vi "Test PWM host.vi"() -> ()   [LabVIEW 2013]
uses:
  <vilib>/userdefined/High Color/nirio_resource_hc.ctl
  <vilib>/rvi/interface/common/niFpgaWaitOnOcc.vi
  <vilib>/FPGAPlugInAG/PCIe-1473R/niLvFpga_Open_PCIe-1473R.vi
  <vilib>/rvi/interface/common/dynamic/niFpgaDynamicAddResources.vi
  <vilib>/Utility/error.llb/Error Cluster From Error Code.vi
  <vilib>/rvi/errors/niLvFpgaAdjustHostInterfaceError.vi
  <vilib>/FPGAPlugInAG/Dynamic/niLvFpga_Close_Dynamic.vi
  <vilib>/rvi/interface/nirviOpenFPGA/nirviOpenFPGA.xnode
  FPGA Bitfiles/PWMTest.lvbitx
  FPGA VIs/PWM FPGA test.vi
  <vilib>/rvi/interface/nirviReadWriteControl/nirviReadWriteControl.xnode
  <vilib>/rvi/interface/nirviCloseFPGA/nirviCloseFPGA.xnode
  NiFpgaLv.dll
  <vilib>/rvi/interface/Simulation/niFpgaSimulationCallBeginRW.vi
panel:
  in  "TTL 1":bool=TRUE
  in  "TTL 2":bool=TRUE
  in  "ISO Out 2":bool
  in  "ISO Out 1":bool
  in  "ISO Out 0":bool
  in  "resource name":T1="rio0" caption="RIO Device"
  out "error out":errorcluster
  out "Running?":bool
  in  "Stop":bool
  in  "Carrier Frequency (Hz)":dbl(slide)=1000.0 scale=0.0..10000000.0 scale format="%#_6p"
  in  "Duty cycle":dbl(slide)=0.5 scale=0.0..1.0
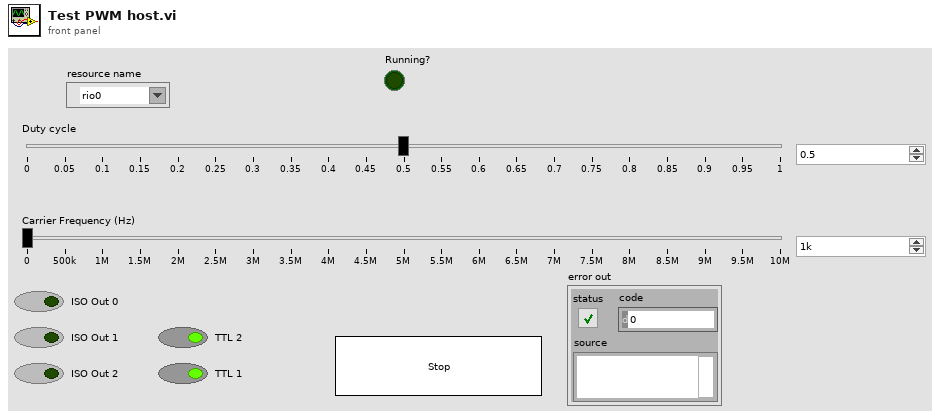
[diagram p1: front panel]
types:
  T1 = typedef "nirio_resource_hc.ctl" = tag
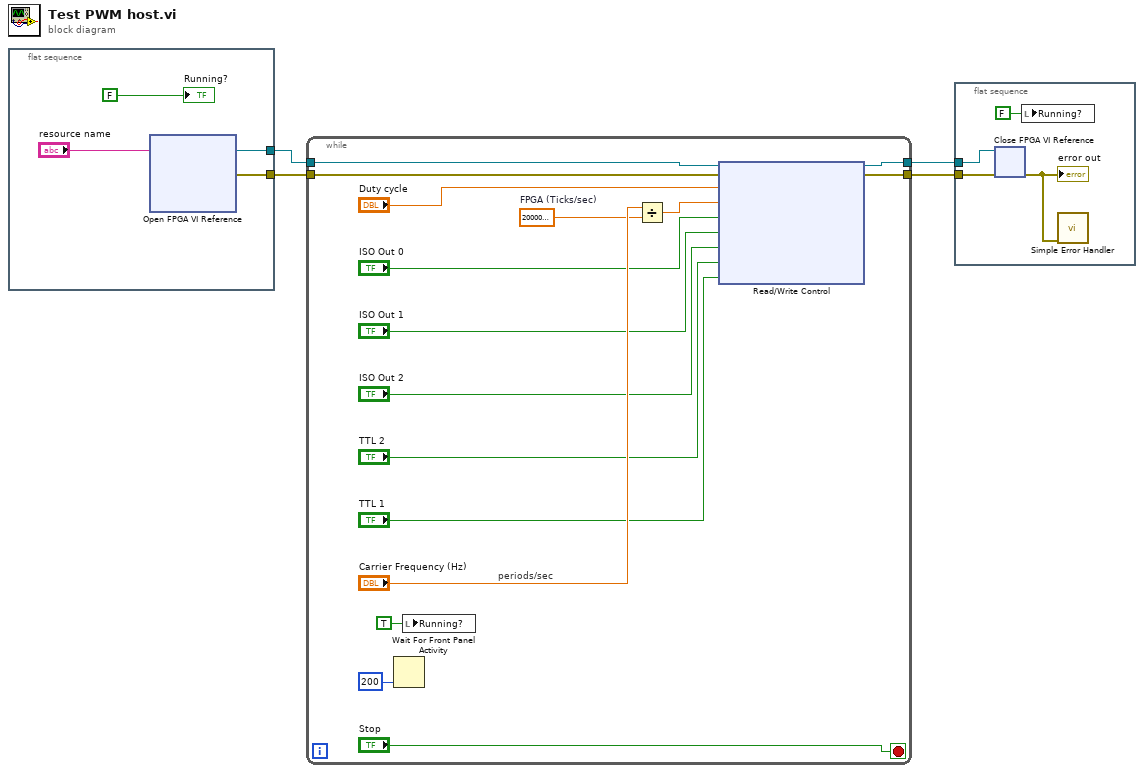
[diagram p0: block diagram]
diagram:
  n1 = flat-sequence {
    tunnel: [w8] -> w4
    tunnel: [w7] -> w3
    frame #0 {
      n2 = xnode "Open FPGA VI Reference"("resource name"="resource name") -> ("FPGA VI Reference Out"=w8:refnum<k20>, "error out"=w7:errorcluster)  [unwired: 1 in]
      "Running?" <- FALSE ("Running?")
    }
  }
  n3 = while {
    tunnel: w4 -> [w24]
    tunnel: w3 -> [w23]
    tunnel: [w18] -> w2
    tunnel: [w17] -> w1
    stop <- "Stop" stop-if-true
    w20 = 200000000.0  # FPGA (Ticks/sec)
    # "periods/sec"
    n4 = Wait For Front Panel Activity(1:200 ("timeout ms (-1 never timeout)")) -> ()  [unwired: 2 in, 1 out]
    n5 = local write "Running?"(TRUE ("Running?")) -> ()
    n6 = Divide(x="Carrier Frequency (Hz)", y=w20) -> (x/y=w19:dbl)
    n7 = xnode "Read/Write Control"("FPGA VI Reference In"=w24, "error in"=w23, "duty cycle (periods)"="Duty cycle", "frequency (periods/tick)"=w19, "ISO Out 0"="ISO Out 0", "ISO Out 1"="ISO Out 1", "ISO Out 2"="ISO Out 2", "TTL 2"="TTL 2", "TTL 1"="TTL 1") -> ("FPGA VI Reference Out"=w17:refnum<k20>, "error out"=w18:errorcluster)
  }
  n8 = flat-sequence {
    tunnel: w2 -> [w28]
    tunnel: w1 -> [w27]
    frame #0 {
      n9 = xnode "Close FPGA VI Reference"("FPGA VI Reference In"=w27, "error in"=w28) -> ("error out"=w25:errorcluster)
      "error out" <- w25
      n10 = local write "Running?"(FALSE ("Running?")) -> ()
      n11 = call <vilib>:"Simple Error Handler.vi"("error in (no error)"=w25) -> ()  [unwired: 4 in, 5 out]
    }
  }
